vi "dfd_Decide Mul Type.vi"(7 "I32 full precision?":T1, 10 "Input wl":i16, 11 "Coef wl":i16) -> (3 "op":T2)   [LabVIEW 2017, in "NI_DigFilter_FXP.lvlib"]
uses:
  <vilib>/addons/Digital Filter Design/NI_DigFilter_FXP.lvlib
  <vilib>/addons/Digital Filter Design/_Objects.llb/dfd_Mul Operation.ctl
  <vilib>/addons/Digital Filter Design/_Objects.llb/DFD FXP MRate Multiply Mode.ctl
  <vilib>/addons/Digital Filter Design/NI_DigFilterLicensed.lvlib
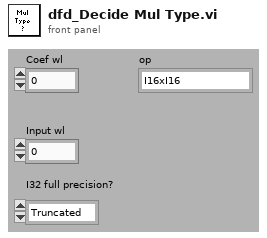
[diagram p1: front panel]
types:
  T1 = typedef "NI_DigFilterLicensed.lvlib/DFD FXP MRate Multiply Mode.ctl" = enum16{"Truncated", "Full"}
  T2 = typedef "dfd_Mul Operation.ctl" = enum16{"I16xI16", "I16xI32", "I32xI16", "I32xI32 (MSBs)", "I32xI32"}
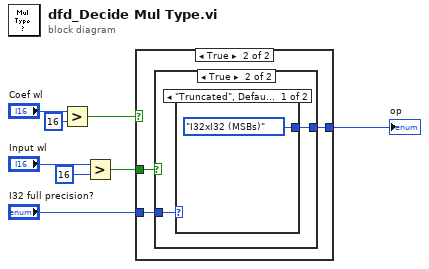
[diagram p0: block diagram]
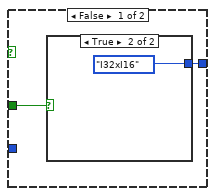
[diagram p2: hidden frame]
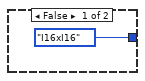
[diagram p3: hidden frame]
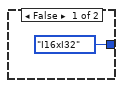
[diagram p4: hidden frame]
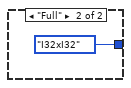
[diagram p5: hidden frame]
diagram:
  n1 = Greater?(x="Coef wl", y=i16 16) -> (0:w5:bool)
  n2 = Greater?(x="Input wl", y=i16 16) -> (0:w2:bool)
  n3 = case shown="True" w5 {
    tunnel: w2 -> [w10 w15]
    tunnel: [w9 w14] -> w8
    tunnel: "I32 full precision?" -> [_ w13]
    frame False {
      n4 = case shown="True" w10 {
        tunnel: [dfd_Mul_Operation."I16xI16" ("op") dfd_Mul_Operation."I32xI16" ("op")] -> w9
        frame False {
        }
        frame True {
        }
      }
    }
    frame True {
      n5 = case shown="True" w15 {
        tunnel: [dfd_Mul_Operation."I16xI32" ("op") w17] -> w14
        tunnel: w13 -> [_ w18]
        frame False {
        }
        frame True {
          n6 = case shown="\"Truncated\", Default" w18 {
            tunnel: [dfd_Mul_Operation."I32xI32 (MSBs)" ("op") dfd_Mul_Operation."I32xI32" ("t")] -> w17
            frame "Truncated", Default {
            }
            frame "Full" {
            }
          }
        }
      }
    }
  }
  "op" <- w8
